vi "生产表头格式.vi"() -> (3 "表头格式":T1)   [LabVIEW 2017]
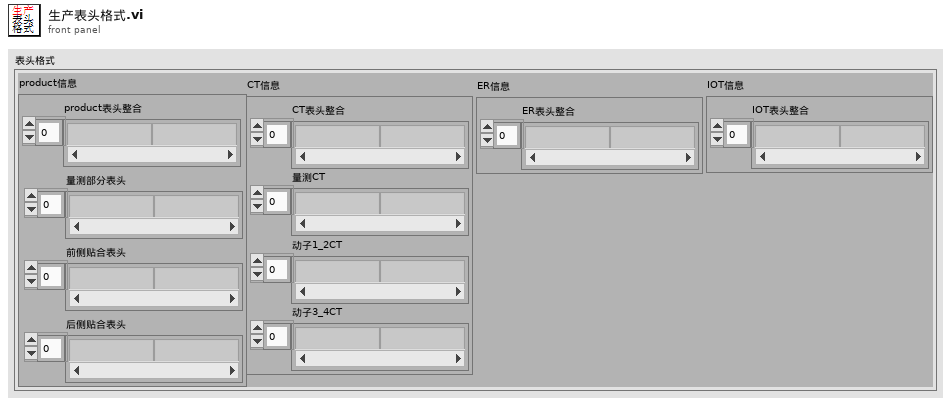
[diagram p1: front panel]
types:
  T1 = typedef "表头集合.ctl" = cluster{"product信息":T2, "CT信息":T3, "ER信息":T4, "IOT信息":T5}
  T2 = typedef "product信息.ctl" = cluster{"product表头整合":string[], "量测部分表头":string[], "前侧贴合表头":string[], "后侧贴合表头":string[]}
  T3 = typedef "CT信息.ctl" = cluster{"CT表头整合":string[], "量测CT":string[], "动子1_2CT":string[], "动子3_4CT":string[]}
  T4 = typedef "ER信息.ctl" = cluster{"ER表头整合":string[]}
  T5 = typedef "IOT信息.ctl" = cluster{"IOT表头整合":string[]}
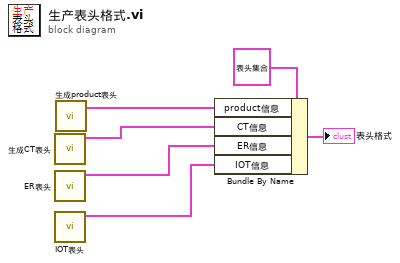
[diagram p0: block diagram]
diagram:
  n1 = call "生成CT表头.vi"() -> ("CT信息"=w3:T3)  [unwired: 11 in]
  n2 = call "ER表头.vi"() -> ("ER信息"=w2:T4)  [unwired: 11 in]
  n3 = call "IOT表头.vi"() -> ("IOT信息"=w1:T5)  [unwired: 11 in]
  n4 = call "生成product表头.vi"() -> ("product信息"=w4:T2)  [unwired: 11 in]
  n5 = Bundle By Name(cluster=T1 {"product信息"={"product表头整合"=[], "量测部分表头"=[], "前侧贴合表头"=[], "后侧贴合表头"=[]}, "CT信息"={"CT表头整合"=[], "量测CT"=[], "动子1_2CT"=[], "动子3_4CT"=[]}, "ER信息"={"ER表头整合"=[]}, "IOT信息"={"IOT表头整合"=[]}} ("表头集合"), "product信息"=w4, "CT信息"=w3, "ER信息"=w2, "IOT信息"=w1) -> (→"表头格式":T1)
